vi "Fpga-MIX_COL.vi"(7 "Tmp":u8, 8 "state[i][y]":u8, 9 "state[i][x]":u8) -> (2 "state[i][x]":u8)   [LabVIEW 2017]
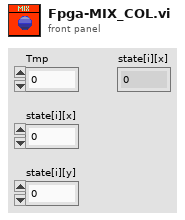
[diagram p1: front panel]
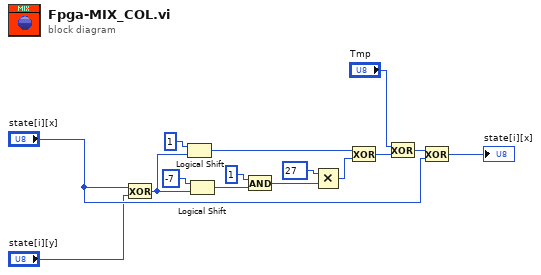
[diagram p0: block diagram]
diagram:
  n1 = Exclusive Or(1:"state[i][y]", 2:"state[i][x]") -> (0:w12:u8)
  n2 = Logical Shift(y=i16 1, x=w12) -> (x << y=w4:u8)
  n3 = Logical Shift(y=i16 -7, x=w12) -> (x << y=w9:u8)
  n4 = And(x=u8 1, y=w9) -> (x .and. y?=w7:u8)
  n5 = Multiply(x=u8 27, y=w7) -> (x*y=w5:u8)
  n6 = Exclusive Or(1:w5, 2:w4) -> (0:w13:u8)
  n7 = Exclusive Or(1:w13, 2:"Tmp") -> (0:w2:u8)
  n8 = Exclusive Or(1:"state[i][x]", 2:w2) -> (0:→"state[i][x]":u8)
